vi "Search File.vi"(8 "error in (no error)":errorcluster, 10 "File/Path Name":string, 11 "Base Path":path) -> (0 "error out":errorcluster, 2 "Full path":path, 3 "Find?":bool)   [LabVIEW 2020, in "Logging.lvlib" / "Logger Mananger.lvclass"]
doc: "search named file or path under base path"
uses:
  Logger Mananger/Logger Mananger.lvclass
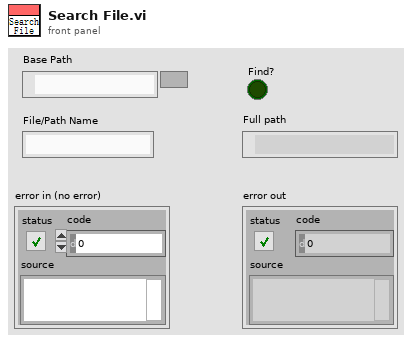
[diagram p1: front panel]
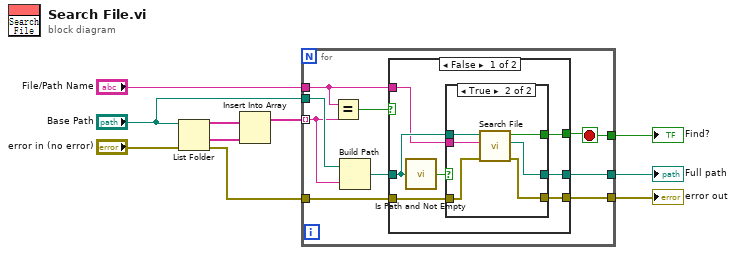
[diagram p0: block diagram]
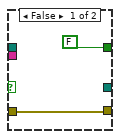
[diagram p2: hidden frame]
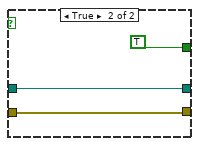
[diagram p3: hidden frame]
diagram:
  n1 = List Folder(path="Base Path", error in="error in (no error)") -> (filenames=w9:string[], folder names=w8:string[], error out=w2:errorcluster)  [unwired: 2 in, 1 out]
  n2 = Insert Into Array(array=w9, new element=w8) -> (w7:string[])  [unwired: 1 in]
  n3 = for {
    tunnel: w7 -> [w15] mode=indexing
    tunnel: "File/Path Name" -> [w13]
    tunnel: "Base Path" -> [w16]
    tunnel: [w18] -> w4
    tunnel: [w14] -> w3
    tunnel: w2 -> [w12]
    tunnel: [w11] -> w1
    stop <- w18 stop-if-true
    n4 = Equal?(x=w13, y=w15) -> (x = y?=w19:bool)
    n5 = Build Path(base path=w16, name or relative path=w15) -> (appended path=w17:path)
    n6 = case shown="False" w19 {
      tunnel: [w25 TRUE] -> w18
      tunnel: w17 -> [w24 w36]
      tunnel: [w22 w36] -> w14
      tunnel: w13 -> [w23 _]
      tunnel: w12 -> [w21 w35]
      tunnel: [w20 w35] -> w11
      frame False {
        n7 = call <vilib>:"Is Path and Not Empty.vi"("path"=w24) -> ("Is Path and Not Empty?"=w26:bool)  [unwired: 4 in]
        n8 = case shown="True" w26 {
          tunnel: [FALSE w34] -> w25
          tunnel: w24 -> [_ w33]
          tunnel: w23 -> [_ w32]
          tunnel: [_ w31] -> w22
          tunnel: w21 -> [w27 w30]
          tunnel: [w27 w29] -> w20
          frame False {
          }
          frame True {
            n9 = call "Search File.vi"("error in (no error)"=w30, "File/Path Name"=w32, "Base Path"=w33) -> ("error out"=w29:errorcluster, "Full path"=w31:path, "Find?"=w34:bool)  [unwired: 6 in]
          }
        }
      }
      frame True {
      }
    }
  }
  "Full path" <- w3
  "error out" <- w1
  "Find?" <- w4
